vi "_attribute_write_string.vi"(5 "Repeated Capability":string, 7 "Attribute":T1={"Identifier"="", "Descriptive Name"="", "Data Type"=enum."Integer 32", "Command"="", "Access"=enum."Read/Write", "Range Table"="", "Read Callback"="", "Write Callback"="", "Supported Models"="", "Instrument Options"="", "Index"=0, "OPC Wait"=FALSE, "No Status Check"=FALSE, "Cache Only"=FALSE}, 8 "error in":errorcluster caption="error in (no error)", 10 "String in":string, 11 "VISA resource name":refnum<visa-resource-name>) -> (0 "error out":errorcluster, 3 "VISA resource name out":refnum<visa-resource-name>)   [LabVIEW 2020, in "Rohde&Schwarz RTx Oscilloscopes.lvlib" / "rsidr_core.lvlib"]
uses:
  rsidr_core.lvlib
  type_Attribute.ctl
  type_Attribute_Data_Type.ctl
  type_ReadWriteAccess.ctl
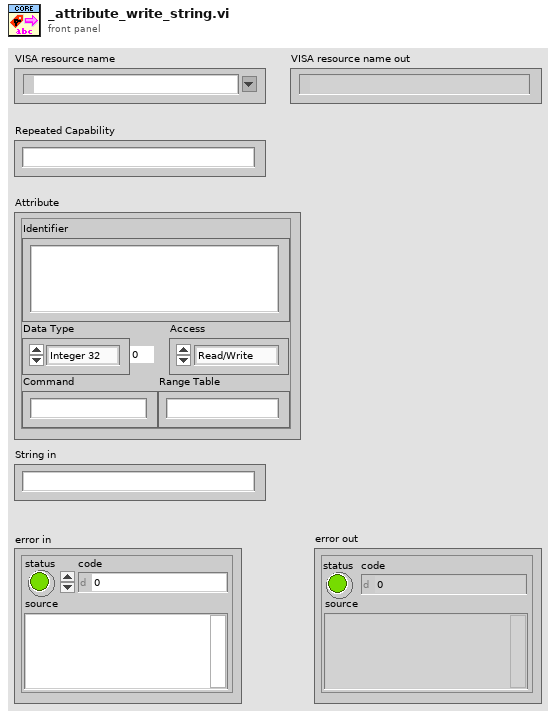
[diagram p1: front panel]
types:
  T1 = typedef "Rohde&Schwarz RTx Oscilloscopes.lvlib/rsidr_core.lvlib/type_Attribute.ctl" = cluster{"Identifier":string, "Descriptive Name":string, "Data Type":T2, "Command":string, "Access":T3, "Range Table":string, "Read Callback":string, "Write Callback":string, "Supported Models":string, "Instrument Options":string, "Index":i32, "OPC Wait":bool, "No Status Check":bool, "Cache Only":bool}
  T2 = typedef "Rohde&Schwarz RTx Oscilloscopes.lvlib/rsidr_core.lvlib/type_Attribute_Data_Type.ctl" = enum16{"Integer 32", "Double", "String", "Boolean", "None", "Integer 64", "RawString"}
  T3 = typedef "Rohde&Schwarz RTx Oscilloscopes.lvlib/rsidr_core.lvlib/type_ReadWriteAccess.ctl" = enum16{"Read Only", "Write Only", "Read/Write"}
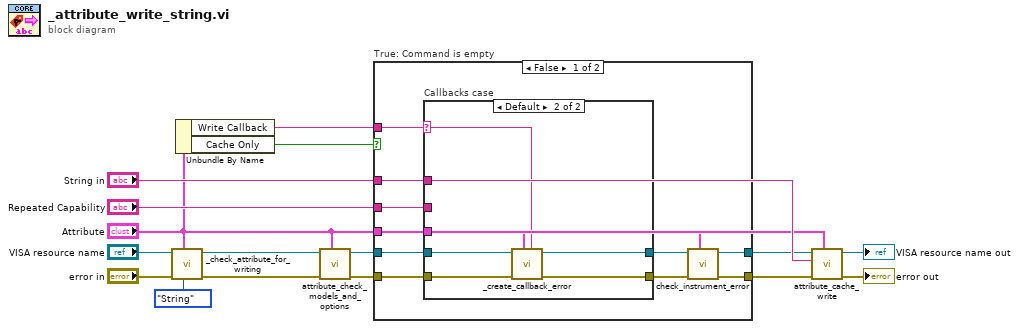
[diagram p0: block diagram]
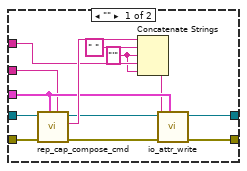
[diagram p2: hidden frame]
diagram:
  n1 = call "_check_attribute_for_writing.vi"("Expected Data Type"=type_Attribute_Data_Type."String" ("Data Type"), "Attribute"="Attribute", "error in"="error in", "VISA resource name"="VISA resource name") -> ("error out"=w7:errorcluster, "VISA resource name out"=w6:refnum<visa-resource-name>)  [unwired: 6 in]
  n2 = Unbundle By Name("Attribute") -> ("Write Callback"=w9:string, "Cache Only"=w1:bool)
  n3 = call "attribute_check_models_and_options.vi"("Attribute"="Attribute", "error in"=w7, "VISA resource name"=w6) -> ("error out"=w5:errorcluster, "VISA resource name out"=w4:refnum<visa-resource-name>)  [unwired: 6 in, 1 out]
  n4 = case "True: Command is empty" shown="False" w1 {
    tunnel: "Repeated Capability" -> [w26 _]
    tunnel: w5 -> [w23 w46]
    tunnel: w4 -> [w22 w47]
    tunnel: "String in" -> [w25 _]
    tunnel: "Attribute" -> [w17 _]
    tunnel: [w18 w47] -> w2
    tunnel: [w19 w46] -> w3
    tunnel: w9 -> [w24 _]
    frame False {
      n5 = case "Callbacks case" shown="Default" w24 {
        selector: w24 -> [_ w40]
        tunnel: w25 -> [w38 _]
        tunnel: w22 -> [w36 w44]
        tunnel: w23 -> [w37 w45]
        tunnel: w26 -> [w30 _]
        tunnel: [w32 w42] -> w20
        tunnel: [w33 w43] -> w21
        tunnel: w17 -> [w31 w41]
        frame "" {
          w28 = "'" ("string")
          n6 = call "rep_cap_compose_cmd.vi"("Repeated Capability"=w30, "Attribute"=w31, "error in"=w37, "VISA resource name"=w36) -> ("error out"=w35:errorcluster, "Command out"=w39:string, "VISA resource name out"=w34:refnum<visa-resource-name>)  [unwired: 5 in]
          n7 = Concatenate Strings(w39, " " ("string"), w28, w38, w28) -> (w27:string)
          n8 = call "io_attr_write.vi"("Attribute"=w31, "error in"=w35, "write buffer"=w27, "VISA resource name"=w34) -> ("error out"=w33:errorcluster, "VISA resource name out"=w32:refnum<visa-resource-name>)  [unwired: 6 in]
        }
        frame Default {
          n9 = call "_create_callback_error.vi"("Callback Name"=w40, "Attribute"=w41, "error in"=w45, "VISA resource name"=w44) -> ("error out"=w43:errorcluster, "VISA resource name out"=w42:refnum<visa-resource-name>)  [unwired: 6 in]
        }
      }
      n10 = call "check_instrument_error.vi"("Attribute"=w17, "error in"=w21, "VISA resource name"=w20) -> ("error out"=w19:errorcluster, "VISA resource name out"=w18:refnum<visa-resource-name>)  [unwired: 7 in]
    }
    frame True {
    }
  }
  n11 = call "attribute_cache_write.vi"("Attribute"="Attribute", "error in"=w3, "Value in"="String in", "VISA resource name"=w2) -> ("error out"=→"error out":errorcluster, "VISA resource name out"=→"VISA resource name out":refnum<visa-resource-name>)  [unwired: 6 in]
